vi "写TDMS文件.vi"() -> ()   [LabVIEW 2010]
doc: "Writes channels of data to different groups in the TDMS file format."
uses:
  Instance           1 18Saved   写TDMS文件 .vi
  Instance           2 18Saved   写TDMS文件 .vi
  Instance           3 18Saved   写TDMS文件 .vi
  Instance           4 18Saved   写TDMS文件 .vi
panel:
  in  "文件路径":path=path "E:/c7/prog7/TDMSFile"
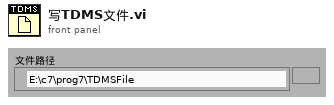
[diagram p1: front panel]
types:
  T1 = enum16{"open", "open or create", "create or replace", "create", "open (read-only)"}
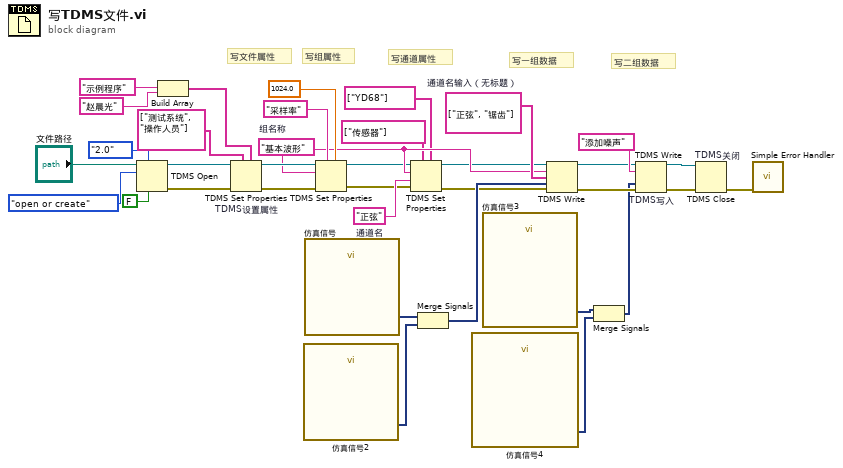
[diagram p0: block diagram]
diagram:
  w9 = "正弦"  # 通道名
  w11 = string[] ["正弦", "锯齿"]  # 通道名输入（无标题）
  w10 = "基本波形"  # 组名称
  # "写二组数据"
  # "写一组数据"
  # "写通道属性"
  # "写组属性"
  # "写文件属性"
  n1 = TDMS Open(6:FALSE ("禁用缓冲？(T)"), 7:enum16{"1.0", "2.0"}."2.0" ("文件格式版本(2.0)"), 10:T1."open or create" ("operation"), 11:"文件路径") -> (0:w16:errorcluster, 3:w17:refnum<k34>)  [unwired: 2 in]
  n2 = Build Array("示例程序" ("name"), "赵晨光" ("元素")) -> (w29:string[])
  n3 = TDMS Set Properties "TDMS设置属性"(5:w29, 7:string[] ["测试系统", "操作人员"] ("property names"), 8:w16, 11:w17) -> (0:w28:errorcluster, 3:w27:refnum<k34>)  [unwired: 2 in, 2 out]
  n4 = call "仿真信号2"() -> ("锯齿波"=w35:dynamicdata)  [unwired: 14 in, 1 out]
  n5 = call "仿真信号"() -> ("正弦"=w34:dynamicdata)  [unwired: 14 in, 1 out]
  n6 = TDMS Set Properties(5:1024.0, 7:"采样率", 8:w28, 10:w10, 11:w27) -> (0:w3:errorcluster, 3:w6:refnum<k34>)  [unwired: 1 in, 2 out]
  n7 = TDMS Set Properties ("TDMS设置属性")(5:string[] ["YD68"], 7:string[] ["传感器"] ("属性名称"), 8:w3, 9:w9, 10:w10, 11:w6) -> (0:w4:errorcluster, 3:w5:refnum<k34>)  [unwired: 2 out]
  n8 = Merge Signals(w34, w35) -> (w25:dynamicdata)
  n9 = call "仿真信号4"() -> ("锯齿波与MLS序列"=w32:dynamicdata)  [unwired: 14 in, 1 out]
  n10 = call "仿真信号3"() -> ("正弦与均匀噪声"=w33:dynamicdata)  [unwired: 14 in, 1 out]
  n11 = TDMS Write ("TDMS写入")(0:w5, 5:w10, 7:w11, 9:w25, 11:w4) -> (4:w23:refnum<k34>, 15:w22:errorcluster)  [unwired: 1 in, 2 out]
  n12 = Merge Signals(w33, w32) -> (w21:dynamicdata)
  n13 = TDMS Write "TDMS写入"(0:w23, 5:"添加噪声", 9:w21, 11:w22) -> (4:w20:refnum<k34>, 15:w19:errorcluster)  [unwired: 2 in, 2 out]
  n14 = TDMS Close "TDMS关闭"(8:w19, 11:w20) -> (0:w15:errorcluster)  [unwired: 1 out]
  n15 = call <vilib>:"Simple Error Handler.vi"("error in (no error)"=w15) -> ()  [unwired: 4 in, 5 out]
